vi "Set ListView Width and Height.vi"(8 "error in (no error)":errorcluster caption="错误输入（无错误）", 9 "Height":i32, 10 "Width":i32, 11 "ListViewClass 输入":refnum<class "ListViewClass.lvclass"> caption="DNL_LabVIEW Object in") -> (0 "error out":errorcluster caption="错误输出", 3 "ListViewClass 输出":refnum<class "ListViewClass.lvclass"> caption="DNL_LabVIEW Object out")   [LabVIEW 2012, in "ListViewClass.lvclass"]
uses:
  ListViewClass.lvclass
  ListViewClass.lvclass/ListViewClass.ctl
  System.Windows.Forms
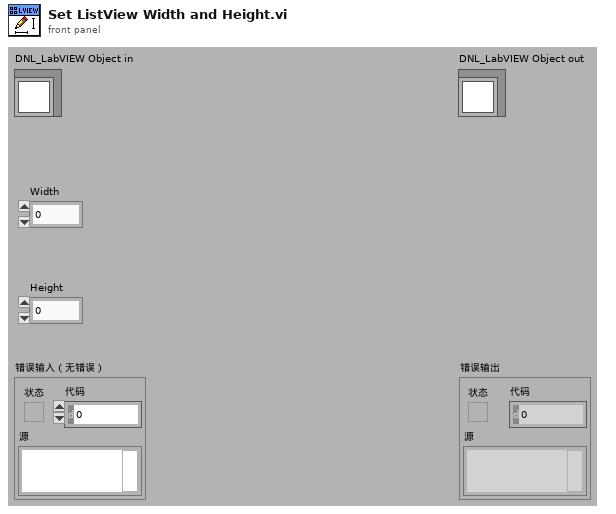
[diagram p1: front panel]
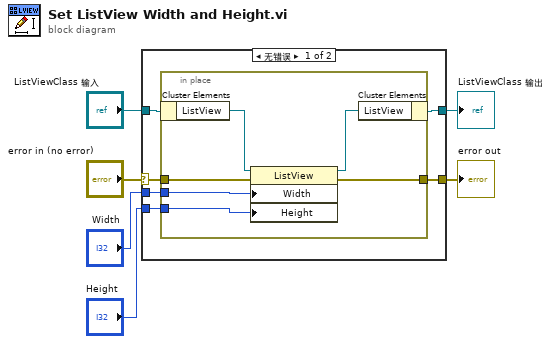
[diagram p0: block diagram]
diagram:
  n1 = case shown="无错误" "error in (no error)" {
    selector: "error in (no error)" -> [w8 w20]
    tunnel: [w7 w20] -> w5
    tunnel: [w9 w19] -> w3
    tunnel: "ListViewClass 输入" -> [w12 w19]
    tunnel: "Width" -> [w11 _]
    tunnel: "Height" -> [w10 _]
    frame No Error {
      n2 = in-place {
        in-place-border: w11 -> [w16]
        in-place-border: w10 -> [w15]
        in-place-border: w8 -> [w14]
        in-place-border: [w13] -> w7
        n3 = in-place-cluster #1(w12) -> ("ListView"=w18:refnum<k24>)
        n4 = property class="ListView"(reference=w18, error in=w14, "Width"=w16, "Height"=w15) -> (reference out=w17:refnum<k24>, error out=w13:errorcluster)
        n5 = in-place-cluster #1("ListView"=w17) -> (w9:refnum<class "ListViewClass.lvclass">)
      }
    }
    frame Error {
    }
  }
  "error out" <- w5
  "ListViewClass 输出" <- w3
